vi "myRIOXC Update State.vi"(8 "error in (no error)":errorcluster, 9 "Display State In":T1, 10 "Facade Ref":refnum<vi>, 11 "Connector Ref":refnum<vi>) -> (0 "error out":errorcluster)   [LabVIEW 2021]
doc: "This VI updates Pin display in xctrl."
uses:
  <vilib>/myRIO/Common/Instrument Driver Framework/Utilities/xctls/utilities/typedefs/myRIOXC Display State.ctl
  <vilib>/regexp/Match Regular Expression.xnode
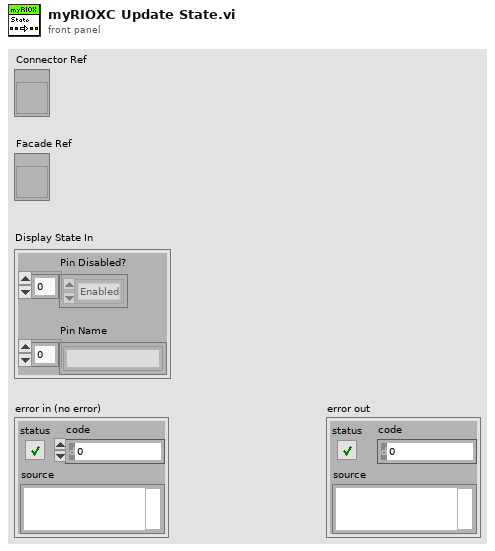
[diagram p1: front panel]
types:
  T1 = typedef "myRIOXC Display State.ctl" = cluster{"Pin Disabled?":enum8{"Enabled", "Disabled", "Disabled and Grayed Out"}[], "Pin Name":string[]}
  T2 = enum8{"Enabled", "Disabled", "Disabled and Grayed Out"}
  T3 = enum8{"Enabled", "Disabled", "Disabled and Grayed Out"}[]
  T4 = typedef "LVFontTypeDef.ctl" = cluster{"Font Name":string, "Size":u16, "Bold":bool, "Italic":bool, "Underline":bool, "Strikeout":bool, "Color":u32}
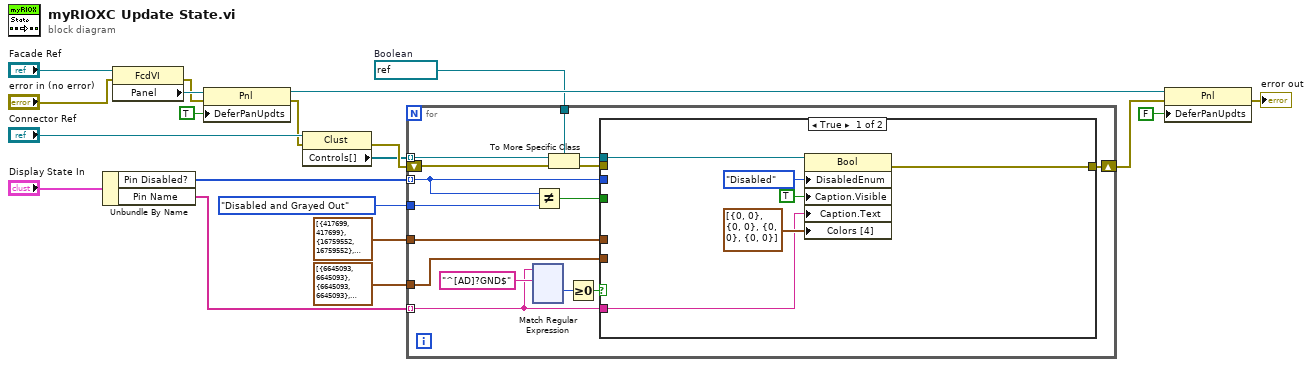
[diagram p0: block diagram]
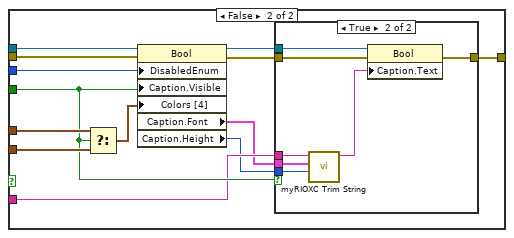
[diagram p2: hidden frame]
diagram:
  w1 = refnum<vi> refnum  # Boolean
  n1 = Unbundle By Name("Display State In") -> ("Pin Disabled?"=w10:T3, "Pin Name"=w5:string[])
  n2 = property class="FcdVI"(reference="Facade Ref", error in="error in (no error)") -> (error out=w19:errorcluster, "Panel"=w20:refnum<vi>)  [unwired: 1 out]
  n3 = property class="Pnl"(reference=w20, error in=w19, "DeferPanUpdts"=TRUE ("Defer Panel Updates")) -> (reference out=w15:refnum<vi>, error out=w8:errorcluster)
  n4 = property class="Clust"(reference="Connector Ref", error in=w8) -> (error out=w7:errorcluster, "Controls[]"=w2:refnum<vi>[])  [unwired: 1 out]
  n5 = for {
    tunnel: w2 -> [w33] mode=indexing
    tunnel: w10 -> [w34] mode=indexing
    shift-right: [w27] -> w14
    shift-left: w7 -> [w26]
    tunnel: T2."Disabled and Grayed Out" ("Disabled") -> [w35]
    tunnel: w5 -> [w21] mode=indexing
    tunnel: w1 -> [w31]
    tunnel: cluster{u32, u32}[] [{6645093, 6645093}, {6645093, 6645093}, {6645093, 6645093}, {6645093, 6645093}] ("Colors [4]") -> [w29]
    tunnel: cluster{u32, u32}[] [{417699, 417699}, {16759552, 16759552}, {208721, 208721}, {8346880, 8346880}] ("Colors [4]") -> [w30]
    n6 = xnode "Match Regular Expression"("input string"=w21, "regular expression"="^[AD]?GND$" ("GND Pattern")) -> ("offset past match"=w23:i32)  [unwired: 4 in, 4 out]
    n7 = Not Equal?(x=w34, y=w35) -> (x != y?=w28:bool)
    n8 = To More Specific Class(target class=w31, reference=w33, error in=w26) -> (specific class reference=w32:refnum<vi>, error out=w25:errorcluster)
    n9 = Greater Or Equal To 0?(x=w23) -> (x >= 0?=w22:bool)
    n10 = case shown="True" w22 {
      tunnel: w34 -> [_ w171]
      tunnel: w32 -> [w158 w170]
      tunnel: w30 -> [_ w168]
      tunnel: w29 -> [_ w167]
      tunnel: w28 -> [_ w166]
      tunnel: w21 -> [w153 w165]
      tunnel: [w157 w162] -> w27
      tunnel: w25 -> [_ w159]
      frame True {
        n11 = property class="Bool"(reference=w158, "DisabledEnum"=T2."Disabled" ("Disabled"), "Caption.Visible"=TRUE, "Caption.Text"=w153, "Colors [4]"=cluster{u32, u32}[] [{0, 0}, {0, 0}, {0, 0}, {0, 0}]) -> (error out=w157:errorcluster)  [unwired: 1 in, 1 out]
      }
      frame False {
        n12 = Select(t=w168, s=w166, f=w167) -> (s? t:f=w169:cluster{u32, u32}[])
        n13 = property class="Bool"(reference=w170, error in=w159, "DisabledEnum"=w171, "Caption.Visible"=w166, "Colors [4]"=w169) -> (reference out=w164:refnum<vi>, error out=w163:errorcluster, "Caption.Font"=w161:T4, "Caption.Height"=w160:u32)
        n14 = case shown="True" w166 {
          tunnel: w161 -> [_ w179]
          tunnel: w165 -> [_ w178]
          tunnel: w164 -> [_ w177]
          tunnel: w160 -> [_ w175]
          tunnel: w163 -> [w172 w174]
          tunnel: [w172 w173] -> w162
          frame False {
          }
          frame True {
            n15 = call <vilib>:"myRIOXC Trim String.vi"("Max Length"=w175, "Text Font"=w179, "Input Text"=w178) -> ("Output Text"=w176:string)  [unwired: 8 in]
            n16 = property class="Bool"(reference=w177, error in=w174, "Caption.Text"=w176) -> (error out=w173:errorcluster)  [unwired: 1 out]
          }
        }
      }
    }
  }
  n17 = property class="Pnl"(reference=w15, error in=w14, "DeferPanUpdts"=FALSE ("Defer Panel Updates")) -> (error out=→"error out":errorcluster)  [unwired: 1 out]
